vi "Initialise OBIS laser.vi"(10 "Laser to initialise":string(combo)) -> (2 "Connected successfully?":bool, 3 "VISA resource name out":refnum<visa-resource-name>)   [LabVIEW 2017]
uses:
  <vilib>/Instr/_visa.llb/VISA Configure Serial Port (Instr).vi
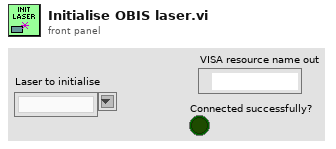
[diagram p1: front panel]
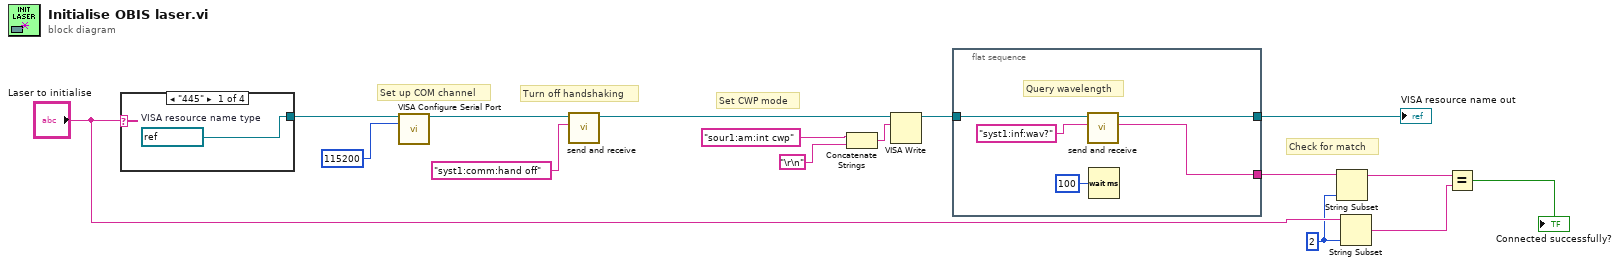
[diagram p0: block diagram]
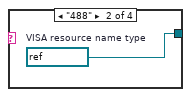
[diagram p2: hidden frame]
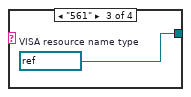
[diagram p3: hidden frame]
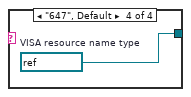
[diagram p4: hidden frame]
diagram:
  w1 = 2 ("length (rest)")
  # "Set CWP mode"
  # "Check for match"
  # "Turn off handshaking"
  # "Set up COM channel"
  n1 = case shown="\"445\"" "Laser to initialise" {
    tunnel: [w17 w18 w19 w20] -> w11
    frame "445" {
      w17 = refnum<visa-resource-name> "COM9"  # VISA resource name type
    }
    frame "488" {
      w18 = refnum<visa-resource-name> "COM8"  # VISA resource name type
    }
    frame "561" {
      w19 = refnum<visa-resource-name> "COM7"  # VISA resource name type
    }
    frame "647", Default {
      w20 = refnum<visa-resource-name> "COM6"  # VISA resource name type
    }
  }
  n2 = call-poly "VISA Configure Serial Port"("VISA resource name"=w11, "baud rate (9600)"=u32 115200) -> ("VISA resource name out"=w15:refnum<visa-resource-name>)  [unwired: 12 in, 1 out]
  n3 = call "send and receive.vi"("write to laser"="syst1:comm:hand off", "VISA resource name"=w15) -> ("VISA resource name out"=w10:refnum<visa-resource-name>)  [unwired: 8 in, 1 out]
  n4 = Concatenate Strings("sour1:am:int cwp", "\r\n") -> (w6:string)
  n5 = VISA Write(VISA resource name=w10, write buffer=w6) -> (VISA resource name out=w9:refnum<visa-resource-name>)  [unwired: 1 in, 2 out]
  n6 = flat-sequence {
    tunnel: [w24] -> w5
    tunnel: w9 -> [w22]
    tunnel: [w21] -> w12
    frame #0 {
      # "Query wavelength"
      n7 = call "send and receive.vi"("write to laser"="syst1:inf:wav?", "VISA resource name"=w22) -> ("read from laser"=w24:string, "VISA resource name out"=w21:refnum<visa-resource-name>)  [unwired: 8 in]
      n8 = Wait (ms)(milliseconds to wait=u32 100) -> ()  [unwired: 1 out]
    }
  }
  n9 = String Subset(string=w5, length (rest)=w1) -> (substring=w2:string)  [unwired: 1 in]
  n10 = String Subset(string="Laser to initialise", length (rest)=w1) -> (substring=w3:string)  [unwired: 1 in]
  n11 = Equal?(x=w2, y=w3) -> (x = y?=→"Connected successfully?":bool)
  "VISA resource name out" <- w12
